vi "Game_Init.vi"(0 "object in":refnum<class "Game.lvclass">, 5 "error in (no error)":errorcluster) -> (14 "object out":refnum<class "Game.lvclass">, 19 "error out":errorcluster)   [LabVIEW 2023, in "Game.lvclass"]
uses:
  Game.lvclass
  Playbook_class/Playbook.lvclass
  Game.lvclass/Game.ctl
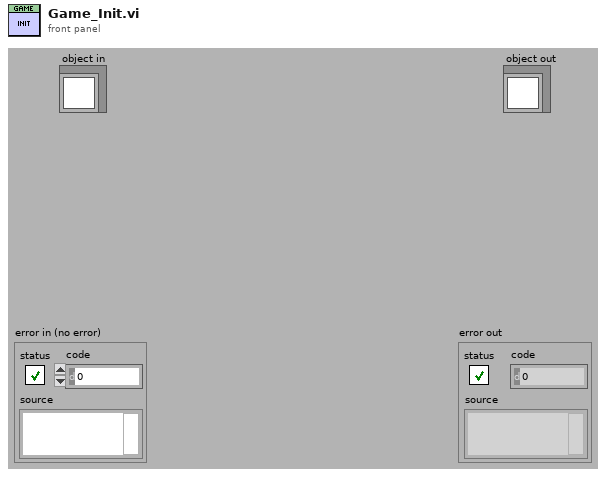
[diagram p1: front panel]
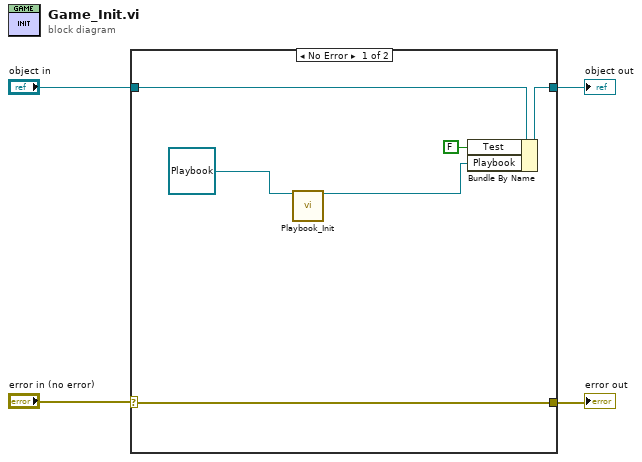
[diagram p0: block diagram]
diagram:
  n1 = case shown="No Error" "error in (no error)" {
    selector: "error in (no error)" -> [w8 w11]
    tunnel: "object in" -> [w10 w12]
    tunnel: [w9 w12] -> w3
    tunnel: [w8 w11] -> w1
    frame No Error {
      n2 = call "Playbook_Init.vi"("object in"=refnum<class "Playbook.lvclass"> refnum ("Playbook")) -> ("object out"=w5:refnum<class "Playbook.lvclass">)  [unwired: 17 in, 1 out]
      n3 = Bundle By Name(cluster=w10, "Test"=FALSE ("None"), "Playbook"=w5) -> (w9:refnum<class "Game.lvclass">)
    }
    frame Error {
    }
  }
  "object out" <- w3
  "error out" <- w1
